vi "TAT_Varient Creater.vi"(8 "error in (no error)":errorcluster) -> (0 "error out":errorcluster)   [LabVIEW 2017]
uses:
  <vilib>/Utility/miscctls.llb/LVRangeTypeDef.ctl
  <vilib>/addons/database/Connection.llb/Conn ObjectReference.ctl
  <vilib>/Utility/miscctls.llb/LVRowAndColumnUnsignedTypeDef.ctl
  b1939813-2d0c-4b6e-8ee7-2e1edd5edc28.vi
  <vilib>/Utility/config.llb/Read Key (I32).vi
  <vilib>/Utility/config.llb/Read Key (String).vi
  <vilib>/Utility/config.llb/Write Key (U32).vi
  <vilib>/Utility/config.llb/Write Key (String).vi
  <vilib>/Utility/config.llb/NI_LVConfig.lvlib
  <vilib>/addons/database/NI_Database_API.lvlib
panel:
  in  "Vertical Slider Control":dbl(slide)=1.0 scale=0.0..-2.0
  in  "CANCLE 3":bool
  in  "PRINTING":bool
  in  "Manual print":bool
  in  "Cancle 2":bool
  in  "Delete Button":bool
  in  "Cancle":bool
  in  "Save Button":bool
  in  "TORISHI CODE":string
  in  "PART NUMBER":string
  in  "Delete Square":bool
  in  "EDIT & SAVE":bool
  out "Varient Details":string[][](table)
  in  "BATCH SIZE":u16=1 min=1 max=100 step=1
  in  "VARIENT NUMBER":u16=1 min=1 max=100 step=1
  in  "HOME":bool
  in  "UPDATE TABLE":bool
  in  "PART NAME":string(combo)
  # "Varient Creater"
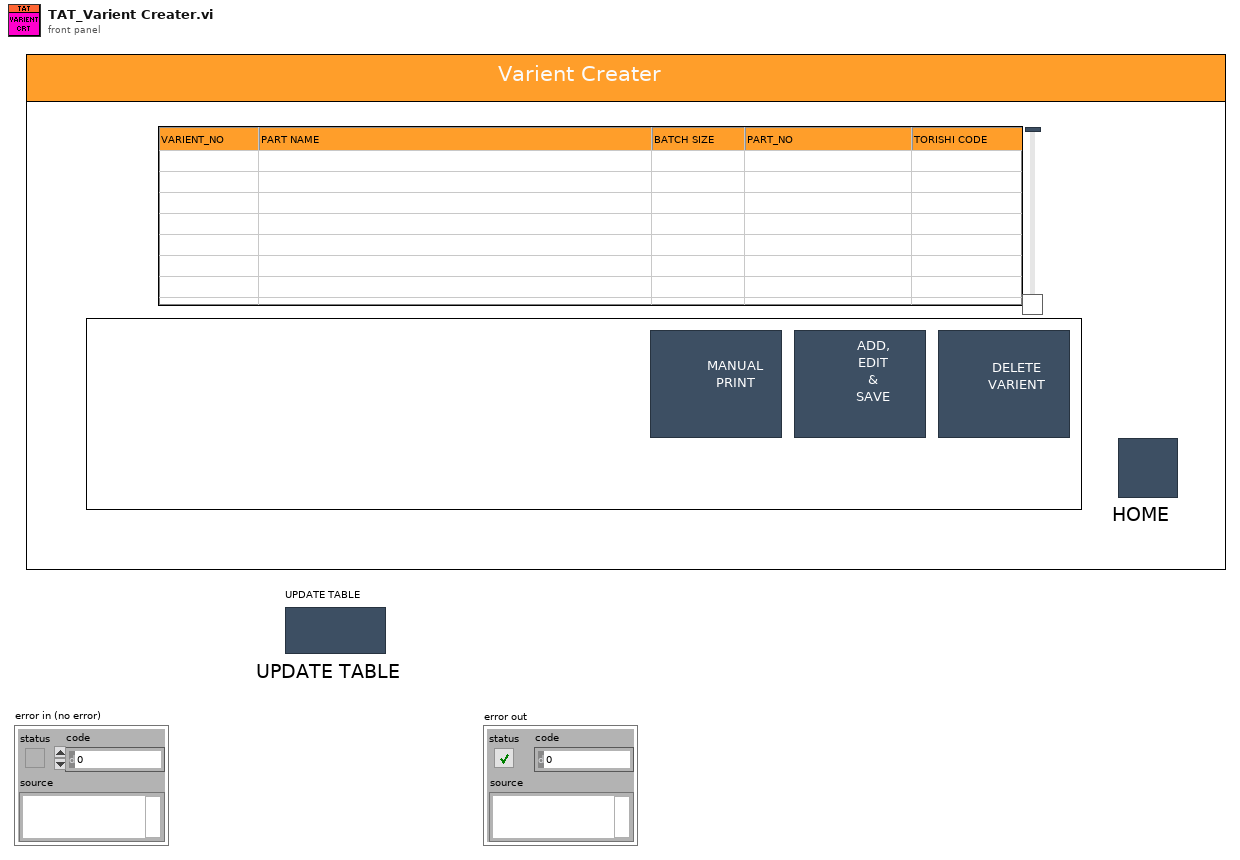
[diagram p1: front panel]
types:
  T1 = enum8{"Enabled", "Disabled", "Disabled and Grayed Out"}
  T2 = enum32{"invalid app kind", "Development System", "Run Time System", "Student Edition", "Embedded LabVIEW", "Evaluation", "Custom"}
  T3 = typedef "NI_LVConfig.lvlib/Config Data RefNum.ctl" = refnum<k1>
  T4 = typedef "LVRangeTypeDef.ctl" = cluster{"Minimum":dbl, "Maximum":dbl, "Increment":dbl, "Minor Increment":dbl, "Start":dbl}
  T5 = typedef "NI_Database_API.lvlib/Conn ObjectReference.ctl" = refnum<k1>
  T6 = cluster{"Varient number":u16, "Part name":string, "connection reference":T5, "Batch_Size":u16, "PART_NO":string, "TORISHI_CODE":string, "scanner com":refnum<visa-resource-name>, "Part Name List":string[], "Varient path":path, "Current Varient path":path, "Communication path":path, "Package path":path, "Part PRN path":path, "Station2 printer IP":string, "Station1 printer IP":string, "Current Serial Number":string, "Station1_QR":string, "Serial_Number":path, "PRIVIOUS code":string[], "Barcode station2 log":string, "Barcode station2 Up":string}
  T7 = typedef "LVRowAndColumnUnsignedTypeDef.ctl" = cluster{"Row":u32, "Column":u32}
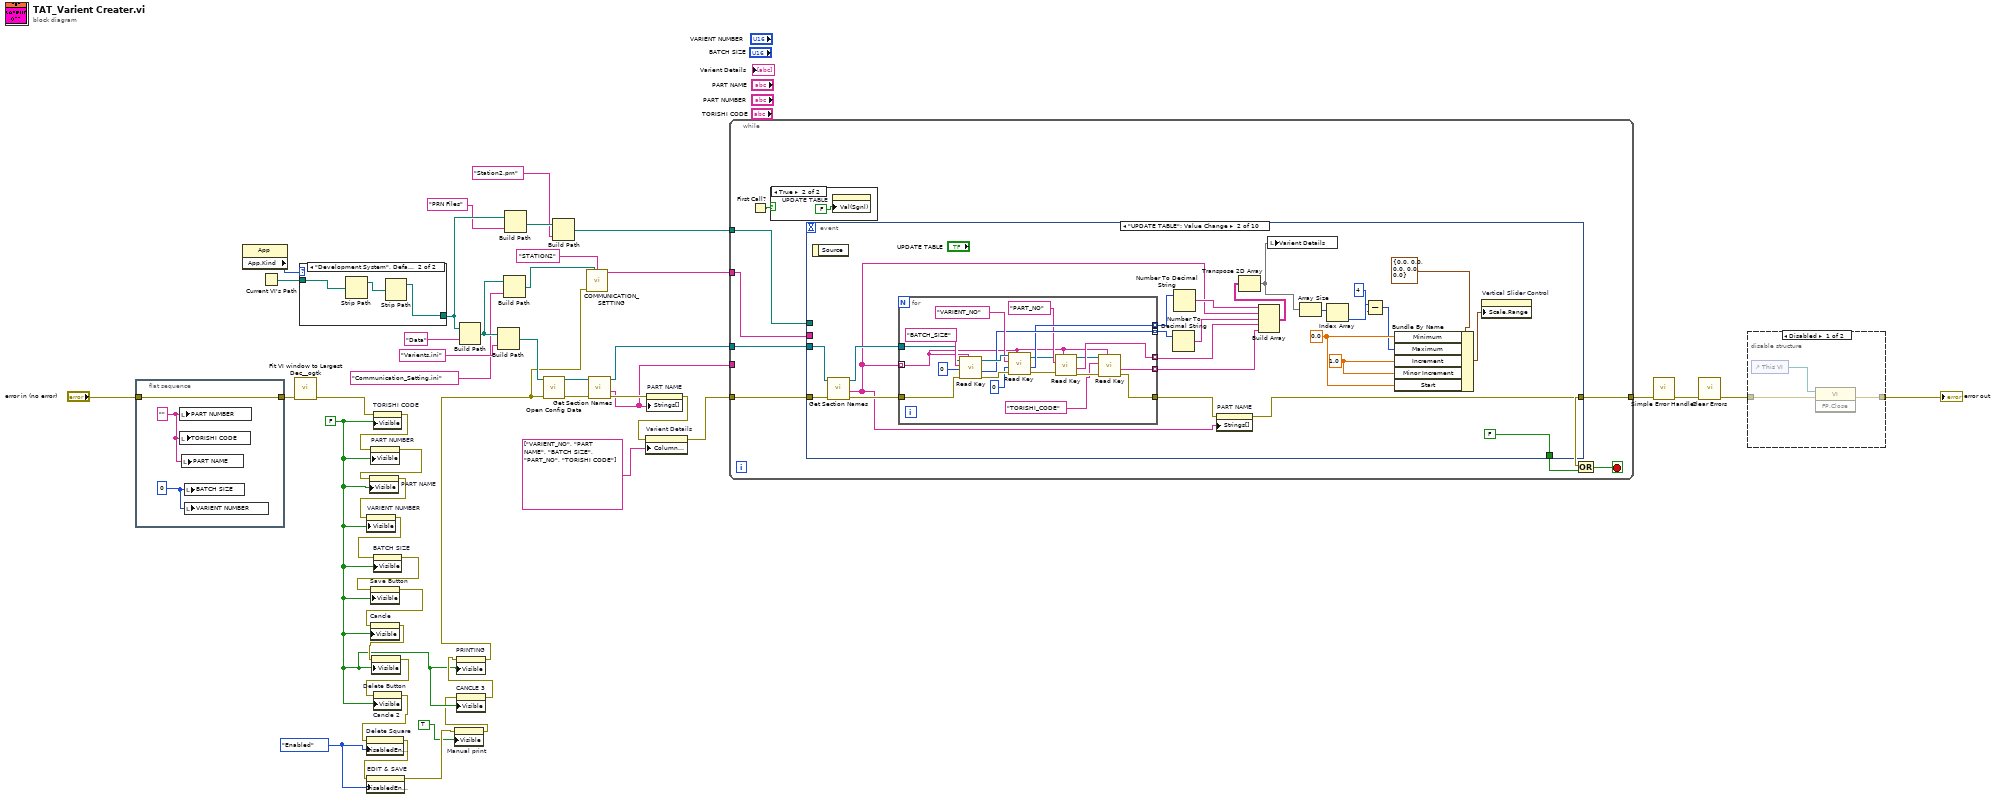
[diagram p0: block diagram]
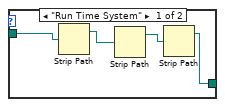
[diagram p3: hidden frame]
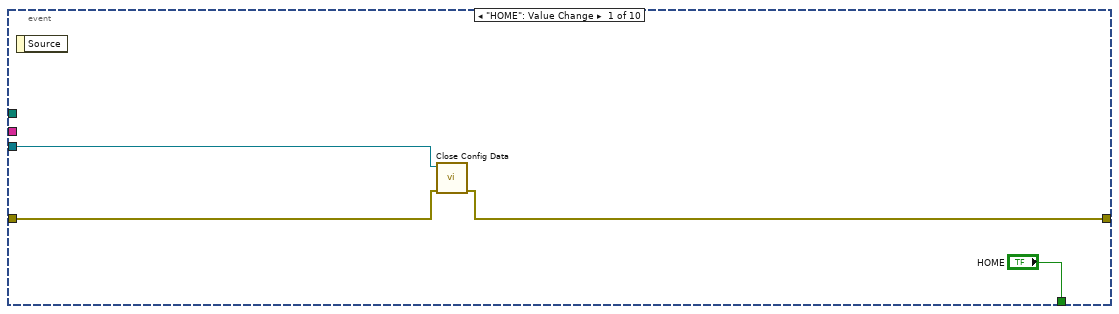
[diagram p5: hidden frame]
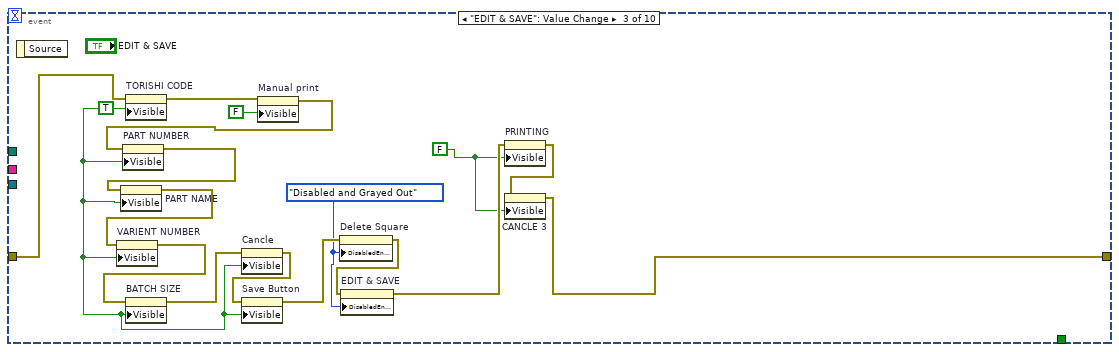
[diagram p6: hidden frame]
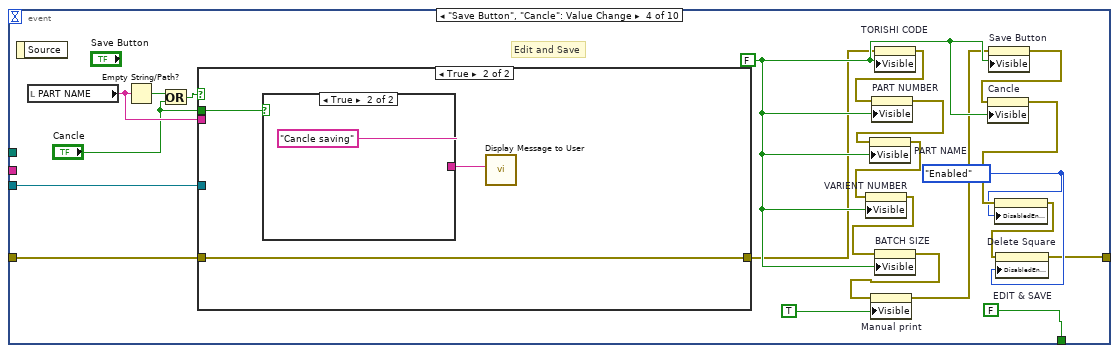
[diagram p7: hidden frame]
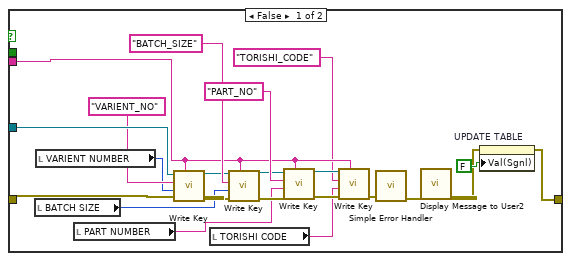
[diagram p8: hidden frame]
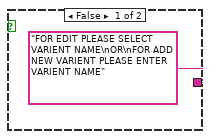
[diagram p9: hidden frame]
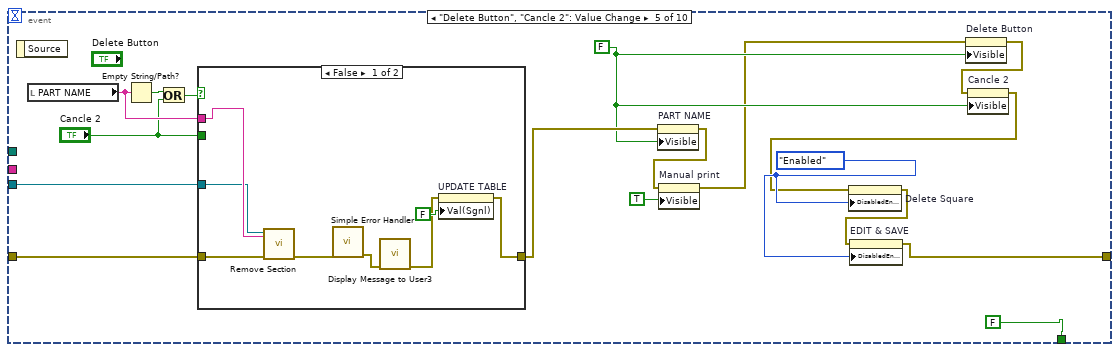
[diagram p10: hidden frame]
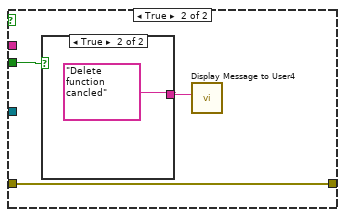
[diagram p11: hidden frame]
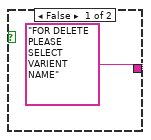
[diagram p12: hidden frame]
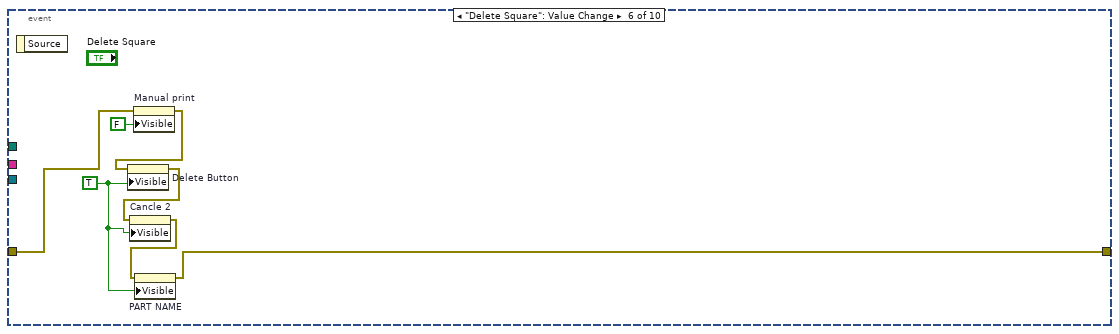
[diagram p13: hidden frame]
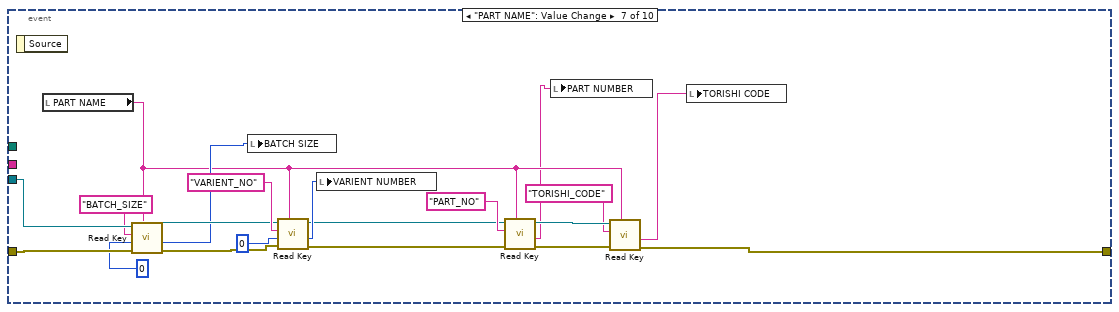
[diagram p14: hidden frame]
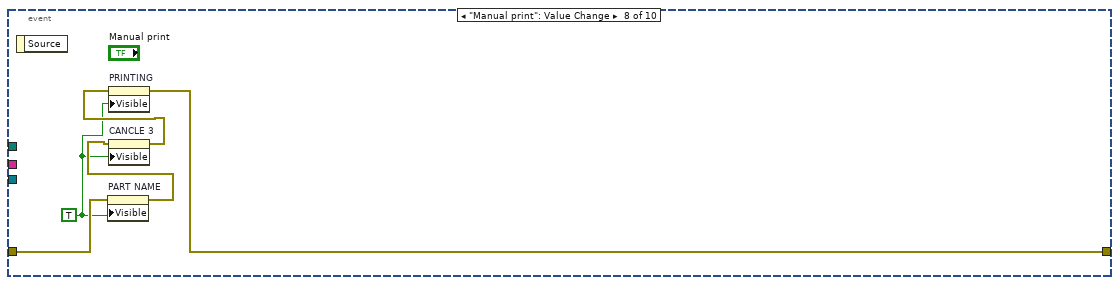
[diagram p15: hidden frame]
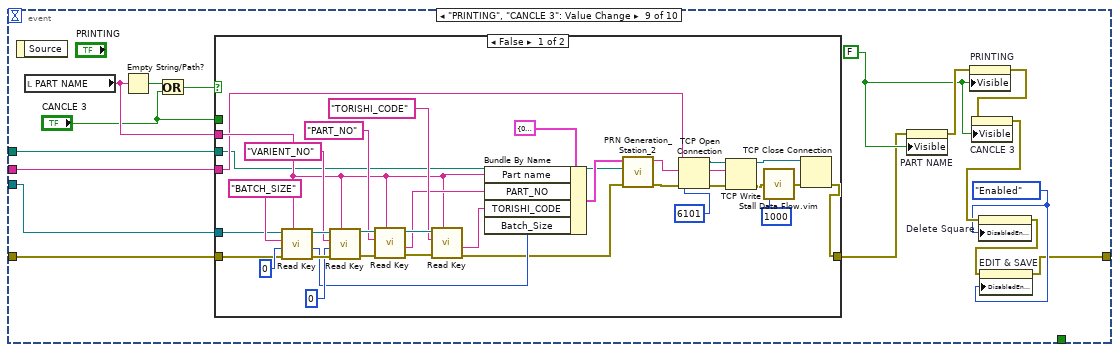
[diagram p16: hidden frame]
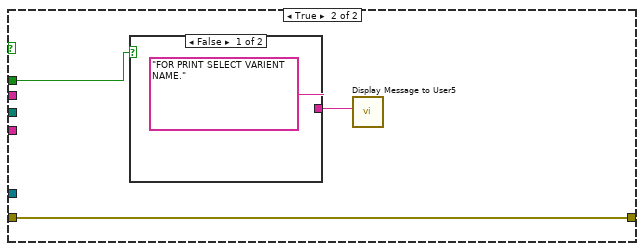
[diagram p17: hidden frame]
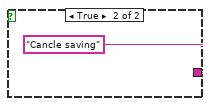
[diagram p18: hidden frame]
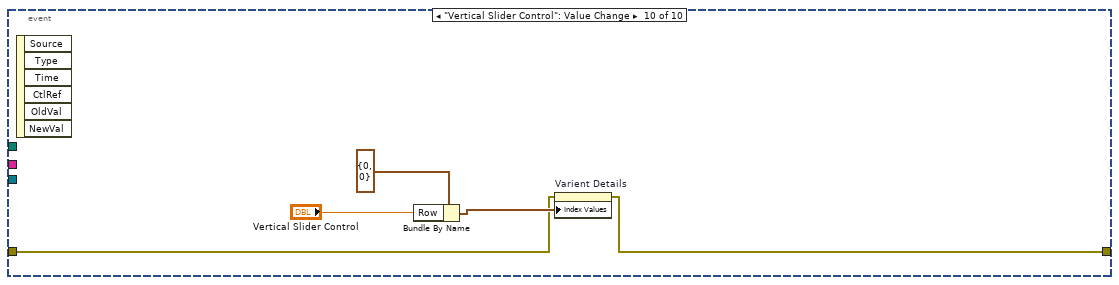
[diagram p19: hidden frame]
diagram:
  w21 = T1."Enabled" ("Disabled")
  w15 = FALSE
  n1 = flat-sequence {
    tunnel: [w48] -> w29
    tunnel: "error in (no error)" -> [w48]
    frame #0 {
      w49 = u16 0 ("BATCH SIZE")
      w50 = "" ("PART NUMBER")
      n2 = local write "PART NUMBER"(w50) -> ()
      n3 = local write "TORISHI CODE"(w50) -> ()
      n4 = local write "PART NAME"(w50) -> ()
      n5 = local write "BATCH SIZE"(w49) -> ()
      n6 = local write "VARIENT NUMBER"(w49) -> ()
    }
  }
  n7 = property class="App"() -> ("App.Kind"=w42:T2)  [unwired: 2 in, 2 out]
  n8 = Current VI's Path() -> (path=w43:path)
  n9 = call <userlib>:"Fit VI window to Largest Dec__ogtk.vi"("error in (no error)"=w29) -> ("error out"=w24:errorcluster)  [unwired: 5 in, 1 out]
  n10 = case shown="\"Development System\", Default" w42 {
    tunnel: w43 -> [w52 w56]
    tunnel: [w51 w55] -> w5
    frame "Run Time System" {
      n11 = Strip Path(path=w52) -> (stripped path=w54:path)  [unwired: 1 out]
      n12 = Strip Path(path=w54) -> (stripped path=w53:path)  [unwired: 1 out]
      n13 = Strip Path(path=w53) -> (stripped path=w51:path)  [unwired: 1 out]
    }
    frame "Development System", Default {
      n14 = Strip Path(path=w56) -> (stripped path=w57:path)  [unwired: 1 out]
      n15 = Strip Path(path=w57) -> (stripped path=w55:path)  [unwired: 1 out]
    }
  }
  n16 = property on="TORISHI CODE" class="Str"(error in=w24, "Visible"=w15) -> (error out=w28:errorcluster)  [unwired: 1 in, 1 out]
  n17 = property on="PART NUMBER" class="Str"(error in=w28, "Visible"=w15) -> (error out=w27:errorcluster)  [unwired: 1 in, 1 out]
  n18 = property on="PART NAME" class="CmbBox"(error in=w27, "Visible"=w15) -> (error out=w26:errorcluster)  [unwired: 1 in, 1 out]
  n19 = property on="VARIENT NUMBER" class="DigNum (strict)"(error in=w26, "Visible"=w15) -> (error out=w25:errorcluster)  [unwired: 1 in, 1 out]
  n20 = property on="BATCH SIZE" class="DigNum (strict)"(error in=w25, "Visible"=w15) -> (error out=w23:errorcluster)  [unwired: 1 in, 1 out]
  n21 = property on="Save Button" class="Bool"(error in=w23, "Visible"=w15) -> (error out=w20:errorcluster)  [unwired: 1 in, 1 out]
  n22 = property on="Cancle" class="Bool"(error in=w20, "Visible"=w15) -> (error out=w19:errorcluster)  [unwired: 1 in, 1 out]
  n23 = property on="Delete Button" class="Bool"(error in=w19, "Visible"=w15) -> (error out=w18:errorcluster)  [unwired: 1 in, 1 out]
  n24 = property on="Cancle 2" class="Bool"(error in=w18, "Visible"=w15) -> (error out=w17:errorcluster)  [unwired: 1 in, 1 out]
  n25 = property on="Delete Square" class="Bool"(error in=w17, "DisabledEnum"=w21) -> (error out=w22:errorcluster)  [unwired: 1 in, 1 out]
  n26 = property on="EDIT & SAVE" class="Bool"(error in=w22, "DisabledEnum"=w21) -> (error out=w14:errorcluster)  [unwired: 1 in, 1 out]
  n27 = property on="Manual print" class="Bool"(error in=w14, "Visible"=TRUE) -> (error out=w13:errorcluster)  [unwired: 1 in, 1 out]
  n28 = property on="CANCLE 3" class="Bool"(error in=w13, "Visible"=w15) -> (error out=w16:errorcluster)  [unwired: 1 in, 1 out]
  n29 = property on="PRINTING" class="Bool"(error in=w16, "Visible"=w15) -> (error out=w7:errorcluster)  [unwired: 1 in, 1 out]
  n30 = Build Path(base path=w5, name or relative path="Data") -> (appended path=w11:path)
  n31 = Build Path(base path=w11, name or relative path="Varients.ini") -> (appended path=w41:path)
  n32 = Build Path(base path=w11, name or relative path="Communication_Setting.ini") -> (appended path=w8:path)
  n33 = Build Path(base path=w5, name or relative path="PRN Files") -> (appended path=w3:path)
  n34 = call <vilib>:"Open Config Data.vi"("error in (no error)"=w7, "configuration file path"=w41) -> ("error out"=w37:errorcluster, "refnum"=w38:T3)  [unwired: 7 in, 1 out]
  n35 = Build Path(base path=w3, name or relative path="Station2.prn") -> (appended path=w1:path)
  n36 = call "COMMUNICATION_SETTING.vi"("communication path"=w8, "error in"=w7, "STATION"="STATION2") -> ("PRINT_COM"=w6:string)  [unwired: 6 in, 2 out]
  n37 = call <vilib>:"Get Section Names.vi"("error in (no error)"=w37, "refnum"=w38) -> ("error out"=w36:errorcluster, "section names"=w31:string[], "refnum out"=w35:T3)  [unwired: 7 in]
  n38 = property on="PART NAME" class="CmbBox"(error in=w36, "Strings[]"=w31) -> (error out=w34:errorcluster)  [unwired: 1 in, 1 out]
  n39 = property on="Varient Details" class="Tbl (strict)"(error in=w34, "Column Headers[]"=string[] ["VARIENT_NO", "PART NAME", "BATCH SIZE", "PART_NO", "TORISHI CODE"] ("Column Header Strings[]")) -> (error out=w33:errorcluster)  [unwired: 1 in, 1 out]
  n40 = while {
    tunnel: w33 -> [w64]
    tunnel: [w62] -> w44
    tunnel: w35 -> [w61]
    tunnel: w31 -> [_]
    tunnel: w6 -> [w59]
    tunnel: w1 -> [w58]
    stop <- w63 stop-if-true
    n41 = First Call?() -> (First Call?: T/F=w60:bool)
    n42 = case shown="True" w60 {
      frame False {
      }
      frame True {
        n43 = property on="UPDATE TABLE" class="Bool (strict)"("Val(Sgnl)"=FALSE) -> ()  [unwired: 2 in, 2 out]
      }
    }
    n44 = event shown="[1] \"UPDATE TABLE\": Value Change" {
      selector: _ -> [_ _ _ _ _ _ _ _ _ _]
      dyn-events: _ -> [_ _ _ _ _ _ _ _ _ _]
      timeout: _ -> [_ _ _ _ _ _ _ _ _ _]
      tunnel: ["HOME" FALSE ("stop") _ FALSE ("stop") FALSE ("stop") _ _ _ _ _] -> w65
      tunnel: w64 -> [w69 w88 w128 w150 w194 w211 w236 w239 w257 w296]
      tunnel: [w68 w80 w116 w135 w186 w214 w223 w238 w246 w297] -> w62
      tunnel: w61 -> [w67 w86 _ w151 w195 _ w235 _ w253 _]
      tunnel: w59 -> [_ _ _ _ _ _ _ _ w244 _]
      tunnel: w58 -> [_ _ _ _ _ _ _ _ w243 _]
      event "HOME": Value Change {
        n45 = event-data() -> ()  [unwired: 1 in, 1 out]
        n46 = call <vilib>:"Close Config Data.vi"("error in (no error)"=w69, "refnum"=w67) -> ("error out"=w68:errorcluster)  [unwired: 8 in, 1 out]
      }
      event "UPDATE TABLE": Value Change {
        w77 = 1.0 ("Increment")
        w76 = 0.0 ("Minimum")
        n47 = event-data() -> ()  [unwired: 1 in, 1 out]
        n48 = call <vilib>:"Get Section Names.vi"("error in (no error)"=w88, "refnum"=w86) -> ("error out"=w87:errorcluster, "section names"=w81:string[], "refnum out"=w85:T3)  [unwired: 7 in]
        n49 = for {
          tunnel: [w99] -> w82
          tunnel: w87 -> [w108]
          tunnel: w81 -> [w96] mode=indexing
          tunnel: w85 -> [w107]
          tunnel: [w106] -> w92 mode=indexing
          tunnel: [w105] -> w93 mode=indexing
          tunnel: [w101] -> w84 mode=indexing
          tunnel: [w95] -> w83 mode=indexing
          n50 = call-poly <vilib>:"Read Key.vi"("section"=w96, "error in (no error)"=w108, "default value"=0, "key"="BATCH_SIZE", "refnum"=w107) -> ("error out"=w114:errorcluster, "value"=w106:i32, "refnum out"=w113:T3)  [unwired: 3 in, 1 out]
          n51 = call-poly <vilib>:"Read Key.vi"("section"=w96, "error in (no error)"=w114, "default value"=0, "key"="VARIENT_NO", "refnum"=w113) -> ("error out"=w104:errorcluster, "value"=w105:i32, "refnum out"=w102:T3)  [unwired: 3 in, 1 out]
          n52 = call-poly <vilib>:"Read Key.vi"("section"=w96, "error in (no error)"=w104, "key"="PART_NO", "refnum"=w102) -> ("error out"=w100:errorcluster, "value"=w101:string, "refnum out"=w98:T3)  [unwired: 4 in, 1 out]
          n53 = call-poly <vilib>:"Read Key.vi"("section"=w96, "error in (no error)"=w100, "key"="TORISHI_CODE", "refnum"=w98) -> ("error out"=w99:errorcluster, "value"=w95:string)  [unwired: 4 in, 2 out]
        }
        n54 = Number To Decimal String(number=w92) -> (decimal integer string=w91:string[])  [unwired: 1 in]
        n55 = Number To Decimal String(number=w93) -> (decimal integer string=w89:string[])  [unwired: 1 in]
        n56 = property on="PART NAME" class="CmbBox"(error in=w82, "Strings[]"=w81) -> (error out=w80:errorcluster)  [unwired: 1 in, 1 out]
        n57 = Build Array(w89, w81, w91, w84, w83) -> (w90:string[][])
        n58 = Transpose 2D Array(2D array=w90) -> (transposed array=w79:string[][])
        n59 = local write "Varient Details"(w79) -> ()
        n60 = Array Size(array=w79) -> (size(s)=w78:i32[])
        n61 = Index Array(array=w78) -> (element=w73:i32)  [unwired: 1 in]
        n62 = Subtract(x=w73, y=4) -> (x-y=w72:i32)
        n63 = Bundle By Name(cluster=T4 {"Minimum"=0.0, "Maximum"=0.0, "Increment"=0.0, "Minor Increment"=0.0, "Start"=0.0} ("Scale.Range"), "Minimum"=w76, "Maximum"=w72, "Increment"=w77, "Minor Increment"=w77, "Start"=w76) -> (w75:T4)
        n64 = property on="Vertical Slider Control" class="Slide (strict)"("Scale.Range"=w75) -> ()  [unwired: 2 in, 2 out]
      }
      event "EDIT & SAVE": Value Change {
        w115 = FALSE
        w125 = T1."Disabled and Grayed Out" ("Disabled")
        w122 = TRUE
        n65 = event-data() -> ()  [unwired: 1 in, 1 out]
        n66 = property on="TORISHI CODE" class="Str"(error in=w128, "Visible"=w122) -> (error out=w121:errorcluster)  [unwired: 1 in, 1 out]
        n67 = property on="Manual print" class="Bool"(error in=w121, "Visible"=FALSE) -> (error out=w120:errorcluster)  [unwired: 1 in, 1 out]
        n68 = property on="PART NUMBER" class="Str"(error in=w120, "Visible"=w122) -> (error out=w129:errorcluster)  [unwired: 1 in, 1 out]
        n69 = property on="PART NAME" class="CmbBox"(error in=w129, "Visible"=w122) -> (error out=w130:errorcluster)  [unwired: 1 in, 1 out]
        n70 = property on="VARIENT NUMBER" class="DigNum (strict)"(error in=w130, "Visible"=w122) -> (error out=w131:errorcluster)  [unwired: 1 in, 1 out]
        n71 = property on="BATCH SIZE" class="DigNum (strict)"(error in=w131, "Visible"=w122) -> (error out=w123:errorcluster)  [unwired: 1 in, 1 out]
        n72 = property on="Cancle" class="Bool"(error in=w123, "Visible"=w122) -> (error out=w124:errorcluster)  [unwired: 1 in, 1 out]
        n73 = property on="Save Button" class="Bool"(error in=w124, "Visible"=w122) -> (error out=w127:errorcluster)  [unwired: 1 in, 1 out]
        n74 = property on="Delete Square" class="Bool"(error in=w127, "DisabledEnum"=w125) -> (error out=w126:errorcluster)  [unwired: 1 in, 1 out]
        n75 = property on="EDIT & SAVE" class="Bool"(error in=w126, "DisabledEnum"=w125) -> (error out=w117:errorcluster)  [unwired: 1 in, 1 out]
        n76 = property on="PRINTING" class="Bool"(error in=w117, "Visible"=w115) -> (error out=w118:errorcluster)  [unwired: 1 in, 1 out]
        n77 = property on="CANCLE 3" class="Bool"(error in=w118, "Visible"=w115) -> (error out=w116:errorcluster)  [unwired: 1 in, 1 out]
      }
      event "Save Button", "Cancle": Value Change {
        w137 = T1."Enabled" ("Disabled")
        w138 = FALSE
        # "Edit and Save"
        n78 = event-data() -> ()  [unwired: 1 in, 1 out]
        n79 = local read "PART NAME"() -> (w149:string)
        n80 = Empty String/Path?(string/path=w149) -> (empty?=w148:bool)
        n81 = Or(x=w148, y="Cancle") -> (x .or. y?=w147:bool)
        n82 = case shown="True" w147 {
          tunnel: w150 -> [w173 w177]
          tunnel: [w167 w177] -> w136
          tunnel: w151 -> [w171 _]
          tunnel: w149 -> [w156 _]
          tunnel: "Cancle" -> [_ w175]
          frame False {
            n83 = local read "BATCH SIZE"() -> (w166:u16)
            n84 = local read "VARIENT NUMBER"() -> (w165:u16)
            n85 = local read "PART NUMBER"() -> (w153:string)
            n86 = call-poly <vilib>:"Write Key.vi"("section"=w156, "error in (no error)"=w173, "value"=w165, "key"="VARIENT_NO", "refnum"=w171) -> ("error out"=w172:errorcluster, "refnum out"=w170:T3)  [unwired: 4 in, 1 out]
            n87 = local read "TORISHI CODE"() -> (w154:string)
            n88 = call-poly <vilib>:"Write Key.vi"("section"=w156, "error in (no error)"=w172, "value"=w166, "key"="BATCH_SIZE", "refnum"=w170) -> ("error out"=w160:errorcluster, "refnum out"=w157:T3)  [unwired: 4 in, 1 out]
            n89 = call-poly <vilib>:"Write Key.vi"("section"=w156, "error in (no error)"=w160, "value"=w153, "key"="PART_NO", "refnum"=w157) -> ("error out"=w161:errorcluster, "refnum out"=w162:T3)  [unwired: 4 in, 1 out]
            n90 = call-poly <vilib>:"Write Key.vi"("section"=w156, "error in (no error)"=w161, "value"=w154, "key"="TORISHI_CODE", "refnum"=w162) -> ("error out"=w159:errorcluster)  [unwired: 4 in, 2 out]
            n91 = call <vilib>:"Simple Error Handler.vi"("error in (no error)"=w159) -> ("error out"=w164:errorcluster)  [unwired: 4 in, 4 out]
            n92 = call "Display Message to User2"("error in (no error)"=w164) -> ("error out"=w163:errorcluster)  [unwired: 9 in, 1 out]
            n93 = property on="UPDATE TABLE" class="Bool (strict)"(error in=w163, "Val(Sgnl)"=FALSE) -> (error out=w167:errorcluster)  [unwired: 1 in, 1 out]
          }
          frame True {
            n94 = case shown="True" w175 {
              tunnel: ["FOR EDIT PLEASE SELECT VARIENT NAME\nOR\nFOR ADD NEW VARIENT PLEASE ENTER VARIENT NAME" "Cancle saving"] -> w176
              frame False {
              }
              frame True {
              }
            }
            n95 = call "Display Message to User"("Message"=w176) -> ()  [unwired: 9 in, 2 out]
          }
        }
        n96 = property on="TORISHI CODE" class="Str"(error in=w136, "Visible"=w138) -> (error out=w145:errorcluster)  [unwired: 1 in, 1 out]
        n97 = property on="PART NUMBER" class="Str"(error in=w145, "Visible"=w138) -> (error out=w144:errorcluster)  [unwired: 1 in, 1 out]
        n98 = property on="PART NAME" class="CmbBox"(error in=w144, "Visible"=w138) -> (error out=w143:errorcluster)  [unwired: 1 in, 1 out]
        n99 = property on="VARIENT NUMBER" class="DigNum (strict)"(error in=w143, "Visible"=w138) -> (error out=w142:errorcluster)  [unwired: 1 in, 1 out]
        n100 = property on="BATCH SIZE" class="DigNum (strict)"(error in=w142, "Visible"=w138) -> (error out=w133:errorcluster)  [unwired: 1 in, 1 out]
        n101 = property on="Manual print" class="Bool"(error in=w133, "Visible"=TRUE) -> (error out=w132:errorcluster)  [unwired: 1 in, 1 out]
        n102 = property on="Save Button" class="Bool"(error in=w132, "Visible"=w138) -> (error out=w140:errorcluster)  [unwired: 1 in, 1 out]
        n103 = property on="Cancle" class="Bool"(error in=w140, "Visible"=w138) -> (error out=w139:errorcluster)  [unwired: 1 in, 1 out]
        n104 = property on="Delete Square" class="Bool"(error in=w139, "DisabledEnum"=w137) -> (error out=w141:errorcluster)  [unwired: 1 in, 1 out]
        n105 = property on="EDIT & SAVE" class="Bool"(error in=w141, "DisabledEnum"=w137) -> (error out=w135:errorcluster)  [unwired: 1 in, 1 out]
      }
      event "Delete Button", "Cancle 2": Value Change {
        w188 = T1."Enabled" ("Disabled")
        w183 = FALSE
        n106 = event-data() -> ()  [unwired: 1 in, 1 out]
        n107 = local read "PART NAME"() -> (w193:string)
        n108 = Empty String/Path?(string/path=w193) -> (empty?=w192:bool)
        n109 = Or(x=w192, y="Cancle 2") -> (x .or. y?=w191:bool)
        n110 = case shown="False" w191 {
          tunnel: w194 -> [w198 w207]
          tunnel: [w203 w207] -> w187
          tunnel: w195 -> [w199 _]
          tunnel: w193 -> [w200 _]
          tunnel: "Cancle 2" -> [_ w206]
          frame False {
            n111 = call <vilib>:"Remove Section.vi"("section"=w200, "error in (no error)"=w198, "refnum"=w199) -> ("error out"=w197:errorcluster)  [unwired: 6 in, 2 out]
            n112 = call <vilib>:"Simple Error Handler.vi"("error in (no error)"=w197) -> ("error out"=w202:errorcluster)  [unwired: 4 in, 4 out]
            n113 = call "Display Message to User3"("error in (no error)"=w202) -> ("error out"=w201:errorcluster)  [unwired: 9 in, 1 out]
            n114 = property on="UPDATE TABLE" class="Bool (strict)"(error in=w201, "Val(Sgnl)"=FALSE) -> (error out=w203:errorcluster)  [unwired: 1 in, 1 out]
          }
          frame True {
            n115 = case shown="True" w206 {
              tunnel: ["FOR DELETE PLEASE SELECT VARIENT NAME" "Delete function cancled"] -> w205
              frame False {
              }
              frame True {
              }
            }
            n116 = call "Display Message to User4"("Message"=w205) -> ()  [unwired: 9 in, 2 out]
          }
        }
        n117 = property on="PART NAME" class="CmbBox"(error in=w187, "Visible"=w183) -> (error out=w181:errorcluster)  [unwired: 1 in, 1 out]
        n118 = property on="Manual print" class="Bool"(error in=w181, "Visible"=TRUE) -> (error out=w180:errorcluster)  [unwired: 1 in, 1 out]
        n119 = property on="Delete Button" class="Bool"(error in=w180, "Visible"=w183) -> (error out=w185:errorcluster)  [unwired: 1 in, 1 out]
        n120 = property on="Cancle 2" class="Bool"(error in=w185, "Visible"=w183) -> (error out=w184:errorcluster)  [unwired: 1 in, 1 out]
        n121 = property on="Delete Square" class="Bool"(error in=w184, "DisabledEnum"=w188) -> (error out=w189:errorcluster)  [unwired: 1 in, 1 out]
        n122 = property on="EDIT & SAVE" class="Bool"(error in=w189, "DisabledEnum"=w188) -> (error out=w186:errorcluster)  [unwired: 1 in, 1 out]
      }
      event "Delete Square": Value Change {
        w213 = TRUE
        n123 = event-data() -> ()  [unwired: 1 in, 1 out]
        n124 = property on="Manual print" class="Bool"(error in=w211, "Visible"=FALSE) -> (error out=w210:errorcluster)  [unwired: 1 in, 1 out]
        n125 = property on="Delete Button" class="Bool"(error in=w210, "Visible"=w213) -> (error out=w216:errorcluster)  [unwired: 1 in, 1 out]
        n126 = property on="Cancle 2" class="Bool"(error in=w216, "Visible"=w213) -> (error out=w215:errorcluster)  [unwired: 1 in, 1 out]
        n127 = property on="PART NAME" class="CmbBox"(error in=w215, "Visible"=w213) -> (error out=w214:errorcluster)  [unwired: 1 in, 1 out]
      }
      event "PART NAME": Value Change {
        n128 = event-data() -> ()  [unwired: 1 in, 1 out]
        n129 = local read "PART NAME"() -> (w219:string)
        n130 = call-poly <vilib>:"Read Key.vi"("section"=w219, "error in (no error)"=w236, "default value"=0, "key"="BATCH_SIZE", "refnum"=w235) -> ("error out"=w232:errorcluster, "value"=w227:i32, "refnum out"=w231:T3)  [unwired: 3 in, 1 out]
        n131 = local write "BATCH SIZE"(w227) -> ()
        n132 = call-poly <vilib>:"Read Key.vi"("section"=w219, "error in (no error)"=w232, "default value"=0, "key"="VARIENT_NO", "refnum"=w231) -> ("error out"=w224:errorcluster, "value"=w230:i32, "refnum out"=w220:T3)  [unwired: 3 in, 1 out]
        n133 = local write "VARIENT NUMBER"(w230) -> ()
        n134 = call-poly <vilib>:"Read Key.vi"("section"=w219, "error in (no error)"=w224, "key"="PART_NO", "refnum"=w220) -> ("error out"=w225:errorcluster, "value"=w218:string, "refnum out"=w226:T3)  [unwired: 4 in, 1 out]
        n135 = local write "PART NUMBER"(w218) -> ()
        n136 = call-poly <vilib>:"Read Key.vi"("section"=w219, "error in (no error)"=w225, "key"="TORISHI_CODE", "refnum"=w226) -> ("error out"=w223:errorcluster, "value"=w217:string)  [unwired: 4 in, 2 out]
        n137 = local write "TORISHI CODE"(w217) -> ()
      }
      event "Manual print": Value Change {
        w237 = TRUE
        n138 = event-data() -> ()  [unwired: 1 in, 1 out]
        n139 = property on="PART NAME" class="CmbBox"(error in=w239, "Visible"=w237) -> (error out=w241:errorcluster)  [unwired: 1 in, 1 out]
        n140 = property on="CANCLE 3" class="Bool"(error in=w241, "Visible"=w237) -> (error out=w240:errorcluster)  [unwired: 1 in, 1 out]
        n141 = property on="PRINTING" class="Bool"(error in=w240, "Visible"=w237) -> (error out=w238:errorcluster)  [unwired: 1 in, 1 out]
      }
      event "PRINTING", "CANCLE 3": Value Change {
        w247 = T1."Enabled" ("Disabled")
        w248 = FALSE
        n142 = event-data() -> ()  [unwired: 1 in, 1 out]
        n143 = local read "PART NAME"() -> (w254:string)
        n144 = Empty String/Path?(string/path=w254) -> (empty?=w256:bool)
        n145 = Or(x=w256, y="CANCLE 3") -> (x .or. y?=w255:bool)
        n146 = case shown="False" w255 {
          tunnel: w257 -> [w279 w293]
          tunnel: [w270 w293] -> w245
          tunnel: w254 -> [w265 _]
          tunnel: w253 -> [w278 _]
          tunnel: w244 -> [w264 _]
          tunnel: w243 -> [w261 _]
          tunnel: "CANCLE 3" -> [_ w291]
          frame False {
            n147 = call-poly <vilib>:"Read Key.vi"("section"=w265, "error in (no error)"=w279, "default value"=0, "key"="BATCH_SIZE", "refnum"=w278) -> ("error out"=w290:errorcluster, "value"=w268:i32, "refnum out"=w289:T3)  [unwired: 3 in, 1 out]
            n148 = call-poly <vilib>:"Read Key.vi"("section"=w265, "error in (no error)"=w290, "default value"=0, "key"="VARIENT_NO", "refnum"=w289) -> ("error out"=w286:errorcluster, "refnum out"=w285:T3)  [unwired: 3 in, 2 out]
            n149 = call-poly <vilib>:"Read Key.vi"("section"=w265, "error in (no error)"=w286, "key"="PART_NO", "refnum"=w285) -> ("error out"=w287:errorcluster, "value"=w266:string, "refnum out"=w288:T3)  [unwired: 4 in, 1 out]
            n150 = call-poly <vilib>:"Read Key.vi"("section"=w265, "error in (no error)"=w287, "key"="TORISHI_CODE", "refnum"=w288) -> ("error out"=w259:errorcluster, "value"=w269:string)  [unwired: 4 in, 2 out]
            n151 = Bundle By Name(cluster=T6 {"Varient number"=0, "Part name"="", "connection reference"=refnum, "Batch_Size"=0, "PART_NO"="", "TORISHI_CODE"="", "scanner com"="", "Part Name List"=[], "Varient path"=path "", "Current Varient path"=path "", "Communication path"=path "", "Package path"=path "", "Part PRN path"=path "", "Station2 printer IP"="", "Station1 printer IP"="", "Current Serial Number"="", "Station1_QR"="", "Serial_Number"=path "", "PRIVIOUS code"=[], "Barcode station2 log"="", "Barcode station2 Up"=""} ("Cluster 2"), "Part name"=w265, "PART_NO"=w266, "TORISHI_CODE"=w269, "Batch_Size"=w268) -> (w263:T6)
            n152 = call "PRN Generation_Station_2.vi"("error in (no error)"=w259, "PRN path"=w261, "Cluster"=w263) -> ("error out"=w258:errorcluster, "PRN to Print"=w260:string)  [unwired: 5 in, 2 out]
            n153 = TCP Open Connection(address=w264, remote port or service name=u16 6101, error in (no error)=w258) -> (connection ID=w275:refnum<k5>, error out=w274:errorcluster)  [unwired: 2 in]
            n154 = TCP Write(connection ID=w275, data in=w260, error in (no error)=w274) -> (connection ID out=w277:refnum<k5>, error out=w273:errorcluster)  [unwired: 1 in, 1 out]
            n155 = call "Stall Data Flow.vim"("value in"=w273, "milliseconds to wait"=u32 1000) -> ("value out"=w276:errorcluster)  [unwired: 1 out]
            n156 = TCP Close Connection(connection ID=w277, error in (no error)=w276) -> (error out=w270:errorcluster)  [unwired: 1 in, 1 out]
          }
          frame True {
            n157 = case shown="False" w291 {
              tunnel: ["FOR PRINT SELECT VARIENT NAME." "Cancle saving"] -> w292
              frame False {
              }
              frame True {
              }
            }
            n158 = call "Display Message to User5"("Message"=w292) -> ()  [unwired: 9 in, 2 out]
          }
        }
        n159 = property on="PART NAME" class="CmbBox"(error in=w245, "Visible"=w248) -> (error out=w252:errorcluster)  [unwired: 1 in, 1 out]
        n160 = property on="PRINTING" class="Bool"(error in=w252, "Visible"=w248) -> (error out=w250:errorcluster)  [unwired: 1 in, 1 out]
        n161 = property on="CANCLE 3" class="Bool"(error in=w250, "Visible"=w248) -> (error out=w249:errorcluster)  [unwired: 1 in, 1 out]
        n162 = property on="Delete Square" class="Bool"(error in=w249, "DisabledEnum"=w247) -> (error out=w251:errorcluster)  [unwired: 1 in, 1 out]
        n163 = property on="EDIT & SAVE" class="Bool"(error in=w251, "DisabledEnum"=w247) -> (error out=w246:errorcluster)  [unwired: 1 in, 1 out]
      }
      event "Vertical Slider Control": Value Change {
        n164 = event-data() -> ()  [unwired: 1 in, 6 out]
        n165 = Bundle By Name(cluster=T7 {"Row"=0, "Column"=0} ("Index Values"), "Row"="Vertical Slider Control") -> (w299:T7)
        n166 = property on="Varient Details" class="Tbl (strict)"(error in=w296, "Index Values"=w299) -> (error out=w297:errorcluster)  [unwired: 1 in, 1 out]
      }
    }
    n167 = Or(x=w62, y=w65) -> (x .or. y?=w63:bool)
  }
  n168 = call <vilib>:"Simple Error Handler.vi"("error in (no error)"=w44) -> ("error out"=w47:errorcluster)  [unwired: 4 in, 4 out]
  n169 = call <vilib>:"Clear Errors.vi"("error in (no error)"=w47) -> ("error out"=w46:errorcluster)  [unwired: 5 in, 1 out]
  n170 = disable-structure shown="Disabled" {
    disable-tunnel: w46 -> [w303 w304]
    disable-tunnel: [w302 w304] -> w45
    frame Disabled {
      n171 = control-ref of="This VI"() -> (w301:refnum<vi>)
      n172 = invoke class="VI" method="FP.Close"(reference=w301, error in=w303) -> (error out=w302:errorcluster)  [unwired: 1 in, 2 out]
    }
    frame Enabled {
    }
  }
  "error out" <- w45
